vi "General-LoadSingleStep.vi"(8 "error in (no error)":errorcluster, 11 "ERP-CreateInstructions in":refnum<class "ERP-CreateInstructions.lvclass">) -> (0 "error out":errorcluster, 2 "Step Number":string, 3 "ERP-CreateInstructions out":refnum<class "ERP-CreateInstructions.lvclass">, 5 "Cluster for Step":T1, 7 "General Process Name":string)   [LabVIEW 2013, in "ERP-CreateInstructions.lvclass"]
uses:
  ERP-CreateInstructions.lvclass
  ERP-CreateInstructions.lvclass/ERP-CreateInstructions.ctl
  <userlib>/_OpenG.lib/string/string.llb/Trim Whitespace (String Array)__ogtk.vi
  <userlib>/_OpenG.lib/array/array.llb/Search 1D Array (String)__ogtk.vi
  <userlib>/_OpenG.lib/array/array.llb/Delete Elements from 1D Array (String)__ogtk.vi
panel:
  out "Step#":i32
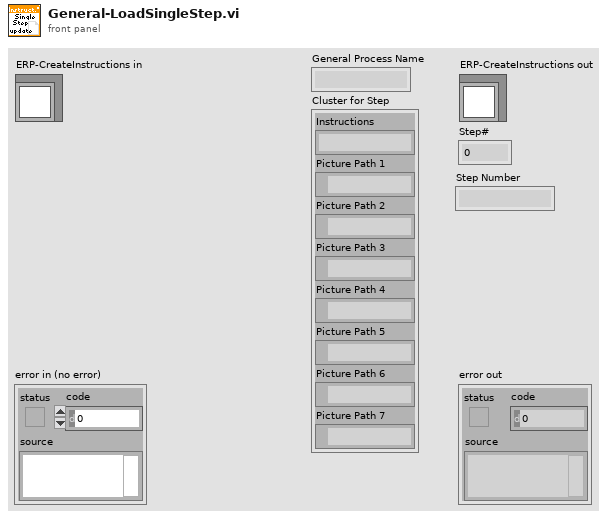
[diagram p1: front panel]
types:
  T1 = cluster{"Instructions":string, "Picture Path 1":path, "Picture Path 2":path, "Picture Path 3":path, "Picture Path 4":path, "Picture Path 5":path, "Picture Path 6":path, "Picture Path 7":path}
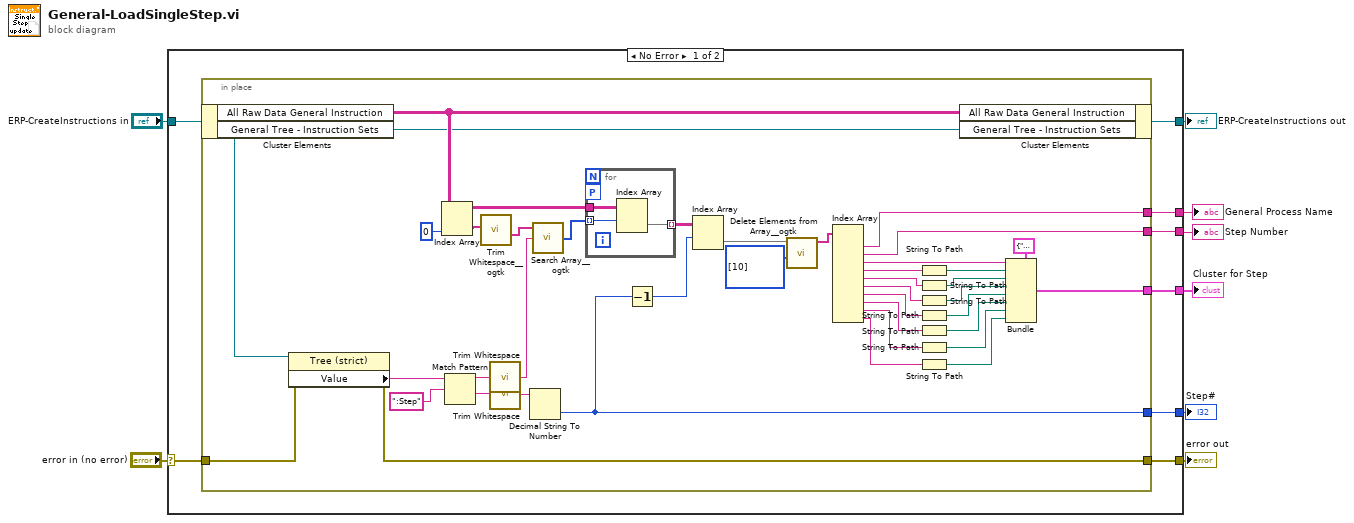
[diagram p0: block diagram]
diagram:
  n1 = case shown="No Error" "error in (no error)" {
    selector: "error in (no error)" -> [w15 w60]
    tunnel: [w13 w60] -> w7
    tunnel: [w16 w59] -> w5
    tunnel: "ERP-CreateInstructions in" -> [w10 w59]
    tunnel: [w14 _] -> w2
    tunnel: [w12 _] -> w4
    tunnel: [w11 _] -> w3
    tunnel: [w9 _] -> w1
    frame No Error {
      n2 = in-place {
        in-place-border: w15 -> [w55]
        in-place-border: [w31] -> w14
        in-place-border: [w41] -> w13
        in-place-border: [w19] -> w12
        in-place-border: [w18] -> w11
        in-place-border: [w17] -> w9
        n3 = in-place-cluster #1(w10) -> ("All Raw Data General Instruction"=w45:string[][], "General Tree - Instruction Sets"=w44:refnum<vi>)
        n4 = property class="Tree (strict)"(reference=w44, error in=w55) -> (error out=w41:errorcluster, "Value"=w54:string)  [unwired: 1 out]
        n5 = Index Array(array=w45, index (col)=0 ("disabled index (col)")) -> (element=w22:string[])  [unwired: 1 in]
        n6 = Match Pattern(string=w54, regular expression=":Step") -> (before substring=w52:string, after substring=w51:string)  [unwired: 1 in, 2 out]
        n7 = call-poly <userlib>:"Trim Whitespace__ogtk.vi"("String in"=w22) -> ("String out"=w21:string[])  [unwired: 6 in]
        n8 = call <vilib>:"Trim Whitespace.vi"("string"=w52) -> ("trimmed string"=w48:string)  [unwired: 1 in]
        n9 = call <vilib>:"Trim Whitespace.vi"("string"=w51) -> ("trimmed string"=w49:string)  [unwired: 1 in]
        n10 = Decimal String To Number(string=w49) -> (number=w19:i32)  [unwired: 2 in, 1 out]
        n11 = call-poly <userlib>:"Search Array__ogtk.vi"("Array"=w21, "Element Data"=w48) -> ("Indices of Elements"=w47:i32[])  [unwired: 7 in]
        n12 = for {
          tunnel: w45 -> [w58]
          tunnel: w47 -> [w57] mode=indexing
          tunnel: [w56] -> w46 mode=indexing
          workers-P: _ -> [_]
          n13 = Index Array(array=w58, index (row)=w57) -> (element=w56:string[])  [unwired: 1 in]
        }
        n14 = Decrement(x=w19) -> (x-1=w20:i32)
        n15 = Index Array(array=w46, index (row)=w20) -> (element=w43:string[])  [unwired: 1 in]
        n16 = call-poly <userlib>:"Delete Elements from Array__ogtk.vi"("indices"=i32[] [10], "array"=w43) -> ("array w/ subset deleted"=w40:string[])  [unwired: 8 in, 1 out]
        n17 = Index Array(array=w40) -> (element #1=w18:string, element #2=w17:string, element #3=w30:string, element #4=w38:string, element #5=w37:string, element #6=w36:string, element #7=w35:string, element #8=w34:string, element #9=w33:string, element #10=w32:string)  [unwired: 10 in]
        n18 = String To Path(string=w38) -> (path=w29:path)
        n19 = String To Path(string=w37) -> (path=w28:path)
        n20 = String To Path(string=w36) -> (path=w27:path)
        n21 = String To Path(string=w35) -> (path=w26:path)
        n22 = String To Path(string=w34) -> (path=w25:path)
        n23 = String To Path(string=w33) -> (path=w24:path)
        n24 = String To Path(string=w32) -> (path=w23:path)
        n25 = in-place-cluster #1("All Raw Data General Instruction"=w45, "General Tree - Instruction Sets"=w44) -> (w16:refnum<class "ERP-CreateInstructions.lvclass">)
        n26 = Bundle(cluster=T1 {"Instructions"="", "Picture Path 1"=path "", "Picture Path 2"=path "", "Picture Path 3"=path "", "Picture Path 4"=path "", "Picture Path 5"=path "", "Picture Path 6"=path "", "Picture Path 7"=path ""}, "Instructions"=w30, "Picture Path 1"=w29, "Picture Path 2"=w28, "Picture Path 3"=w27, "Picture Path 4"=w26, "Picture Path 5"=w25, "Picture Path 6"=w24, "Picture Path 7"=w23) -> (w31:T1)
      }
    }
    frame Error {
    }
  }
  "error out" <- w7
  "ERP-CreateInstructions out" <- w5
  "Step#" <- w4
  "General Process Name" <- w3
  "Cluster for Step" <- w2
  "Step Number" <- w1
